vi "construct.vi"(8 "error in (no error)":errorcluster, 9 "configuration name":string, 10 "load config file?":bool=TRUE, 11 "DL090202FPGAClock in":refnum<class "ClockDL090202FPGA.lvclass">) -> (0 "error out":errorcluster, 3 "DL090202FPGAClock out":refnum<class "ClockDL090202FPGA.lvclass">)   [LabVIEW 2010, in "ClockDL090202FPGA.lvclass"]
uses:
  ClockDL090202FPGA.lvclass
  GenericClock/GenericClock/GenericClock.lvclass
  ClockDL090202FPGA.lvclass/ClockDL090202FPGA.ctl
  common/classes/ErrorController/ErrorController/class_data.vi
  common/classes/ErrorController/ErrorController/ErrorController.lvclass
  common/classes/GenericComponent/GenericComponent/GenericComponent.lvclass
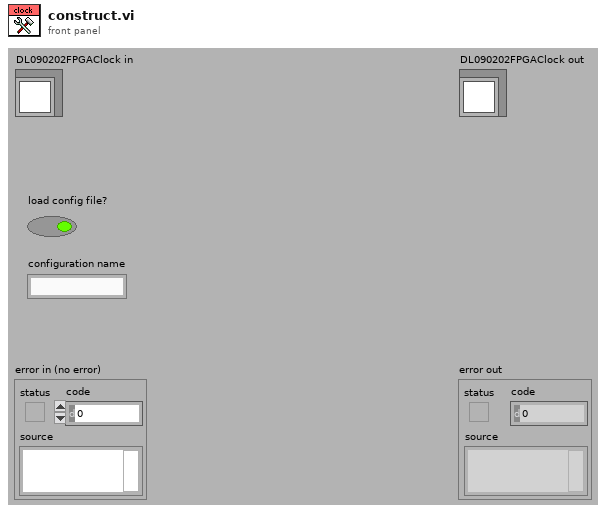
[diagram p1: front panel]
types:
  T1 = typedef "plugin_specification.ctl" = cluster{"class path":string, "configuration":string, "label":string, "settings name":string}
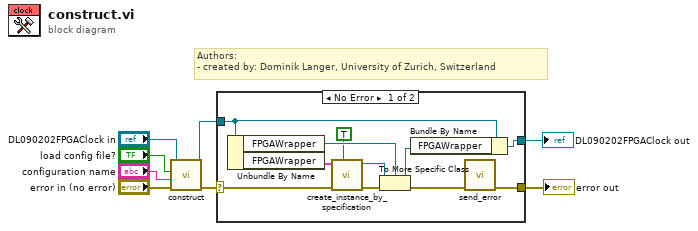
[diagram p0: block diagram]
diagram:
  # "Authors: \n- created by: Dominik Langer, University of Zurich, Switzerland"
  n1 = call-parent "construct.vi"("error in (no error)"="error in (no error)", "configuration name"="configuration name", "load config file?"="load config file?", "GenericPlugin in"="DL090202FPGAClock in") -> ("error out"=w4:errorcluster, "GenericPlugin out"=w3:refnum<class "ClockDL090202FPGA.lvclass">)  [unwired: 6 out]
  n2 = case shown="No Error" w4 {
    selector: w4 -> [w16 w21]
    tunnel: w3 -> [w19 w20]
    tunnel: [w17 w21] -> w2
    tunnel: [w18 w20] -> w1
    frame No Error {
      n3 = Unbundle By Name(w19) -> ("FPGAWrapper"=w12:refnum<class "GenericFPGAWrapper.lvclass">, "FPGAWrapper"=w13:T1)
      n4 = call "create_instance_by_specification.vi"("call constructor?"=TRUE, "error in (no error)"=w16, "component specification"=w13) -> ("error out"=w15:errorcluster, "GenericPlugin out"=w14:refnum<class "GenericComponent.lvclass">)  [unwired: 6 in, 1 out]
      n5 = To More Specific Class(target class=w12, reference=w14, error in=w15) -> (specific class reference=w10:refnum<class "GenericFPGAWrapper.lvclass">, error out=w11:errorcluster)
      n6 = Bundle By Name(cluster=w19, "FPGAWrapper"=w10) -> (w18:refnum<class "ClockDL090202FPGA.lvclass">)
      n7 = call "send_error.vi"("error in (no error)"=w11) -> ("error out"=w17:errorcluster)  [unwired: 10 in]
    }
    frame Error {
    }
  }
  "error out" <- w2
  "DL090202FPGAClock out" <- w1
